vi "IPS magnet power supply - Init.vi"(8 "error in (no error)":errorcluster) -> (0 "error out":errorcluster, 3 "VISA resource name out":refnum<visa-resource-name>)   [LabVIEW 2019]
uses:
  _Global variables 1.vi
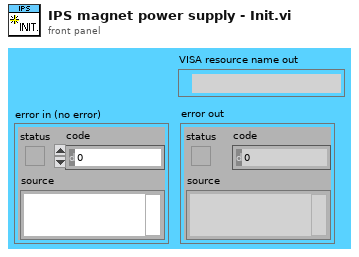
[diagram p1: front panel]
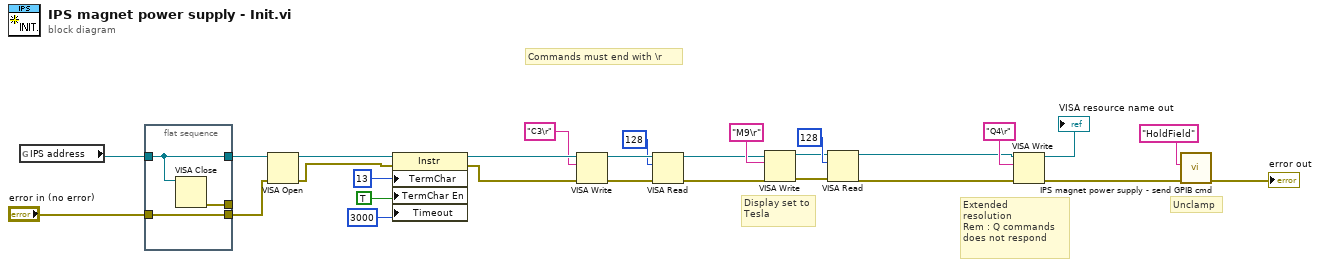
[diagram p0: block diagram]
diagram:
  # "Unclamp"
  # "Display set to\nTesla"
  # "Extended\nresolution\nRem : Q commands\ndoes not respond"
  # "Commands must end with \\r"
  n1 = global read "_Global variables 1.vi" "IPS address"() -> (w2:refnum<visa-resource-name>)
  n2 = flat-sequence {
    tunnel: w2 -> [w30]
    tunnel: "error in (no error)" -> [w31]
    tunnel: [w31] -> w3
    tunnel: [w30] -> w1
    tunnel: [w29] -> _
    frame #0 {
      n3 = VISA Close(VISA resource name=w30) -> (error out=w29:errorcluster)  [unwired: 1 in]
    }
  }
  n4 = VISA Open(error in (no error)=w3, VISA resource name=w1) -> (VISA resource name=w6:refnum<visa-resource-name>, error out=w5:errorcluster)  [unwired: 3 in]
  n5 = property class="Instr"(reference=w6, error in=w5, "TermChar"=u8 13 ("Message Based Settings:Termination Character"), "TermChar En"=TRUE ("Message Based Settings:Termination Character Enable"), "Timeout"=u32 3000 ("General Settings:Timeout Value")) -> (reference out=w12:refnum<visa-resource-name>, error out=w11:errorcluster)
  n6 = VISA Write(VISA resource name=w12, write buffer="C3\r" ("Write Buffer"), error in (no error)=w11) -> (VISA resource name out=w9:refnum<visa-resource-name>, error out=w8:errorcluster)  [unwired: 1 out]
  n7 = VISA Read(VISA resource name=w9, byte count=u32 128, error in (no error)=w8) -> (VISA resource name out=w20:refnum<visa-resource-name>, error out=w19:errorcluster)  [unwired: 2 out]
  n8 = VISA Write(VISA resource name=w20, write buffer="M9\r" ("Write Buffer"), error in (no error)=w19) -> (VISA resource name out=w22:refnum<visa-resource-name>, error out=w23:errorcluster)  [unwired: 1 out]
  n9 = VISA Read(VISA resource name=w22, byte count=u32 128, error in (no error)=w23) -> (VISA resource name out=w18:refnum<visa-resource-name>, error out=w17:errorcluster)  [unwired: 2 out]
  n10 = VISA Write(VISA resource name=w18, write buffer="Q4\r" ("Write Buffer"), error in (no error)=w17) -> (VISA resource name out=→"VISA resource name out":refnum<visa-resource-name>, error out=w16:errorcluster)  [unwired: 1 out]
  n11 = call "IPS magnet power supply - send GPIB cmd.vi"("error in (no error)"=w16, "Cmd string"="HoldField") -> ("error out"=→"error out":errorcluster)  [unwired: 8 in, 1 out]
